vi "svx_Oct_Scale Num Plots.vi"(7 "Display State In":T1={"X Scale Width %"=50.0, "Y Scale Height %"=50.0, "X-Axis Range"={"Minimum"=0.0, "Maximum"=10.0}, "Y-Axis Range"={"Minimum"=0.0, "Maximum"=10.0}, "Z-Axis Range"={"Minimum"=0.0, "Maximum"=10.0}, "Plot Color"=0, "Frame Color"=61212, "Background Color"=16252785, "Initial AutoScale Y"=TRUE, "AutoScale X"=2, "AutoScale Y"=2, "AutoScale Z"=2, "Plot Transparency"=FALSE, "X-Axis Name"="Frequency", "Y-Axis Name"="Amplitude", "Z-Axis Name"="", "X-Axis Scaling Factor"={"Offset"=0.0, "Multiplier"=1.0}, "Y-Axis Scaling Factor"={"Offset"=0.0, "Multiplier"=1.0}, "Z-Axis Scaling Factor"={"Offset"=0.0, "Multiplier"=1.0}, "X-Scale Visible"=TRUE, "Y-Scale Visible"=TRUE, "Z-Scale Visible"=TRUE, "X-Scale Label Visible"=TRUE, "Y-Scale Label Visible"=TRUE, "Z-Scale Label Visible"=TRUE, "X-Axis Range Scaled"={"Minimum"=0.0, "Maximum"=10.0}, "Y-Axis Range Scaled"={"Minimum"=0.0, "Maximum"=10.0}, "Z-Axis Range Scaled"={"Minimum"=0.0, "Maximum"=10.0}, "Rev Z Order"=FALSE, "X-Scale Format Str"="%#.4g", "Y-Scale Format Str"="%#.4g", "Z-Scale Format Str"="%#.4g", "Decor color"=12369084, "Scale Range Change"=refnum, "out of state queue"=refnum, "property nodes"=refnum} caption="State", 11 "Waveform Array In":T2={"z0"=0.0, "dz"=1.0, "Plots"=[]} {"Plots"."Y" format="%.2f"; "Plots"."X" format="%.2f"}) -> (1 "Z length":i32, 2 "Z Index":i32, 3 "Waveform Array Out":T2={"z0"=0.0, "dz"=1.0, "Plots"=[]} {"Plots"."Y" format="%.2f"; "Plots"."X" format="%.2f"})   [LabVIEW 2017, in "SVX Octave Waterfall Graph.xctl"]
uses:
  <vilib>/addons/_XControls/Octave Waterfall Graph/SVX Octave Waterfall Graph.xctl
  <vilib>/addons/_XControls/Octave Waterfall Graph/subVIs/svx_Oct_Waterfall Data.ctl
  <vilib>/addons/_XControls/Octave Waterfall Graph/subVIs/svx_Oct_Waterfall State.ctl
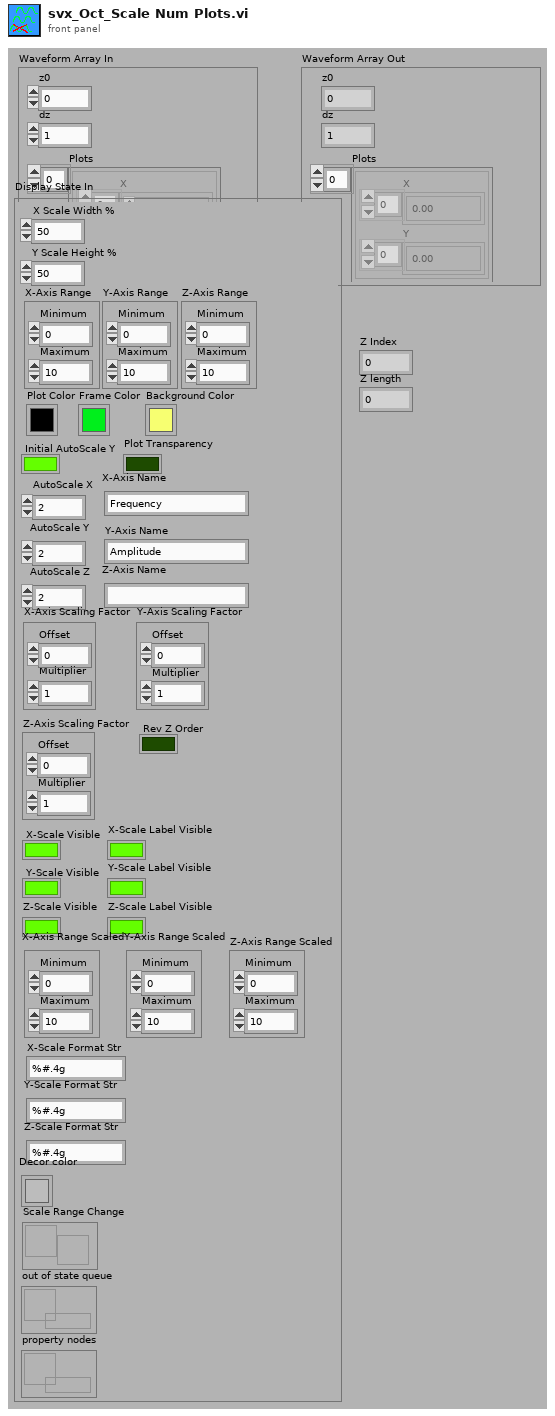
[diagram p1: front panel]
types:
  T1 = typedef "SVX Octave Waterfall Graph.xctl/svx_Oct_Waterfall State.ctl" = cluster{"X Scale Width %":dbl, "Y Scale Height %":dbl, "X-Axis Range":cluster{"Minimum":dbl, "Maximum":dbl}, "Y-Axis Range":cluster{"Minimum":dbl, "Maximum":dbl}, "Z-Axis Range":cluster{"Minimum":dbl, "Maximum":dbl}, "Plot Color":u32, "Frame Color":u32, "Background Color":u32, "Initial AutoScale Y":bool, "AutoScale X":u8, "AutoScale Y":u8, "AutoScale Z":u8, "Plot Transparency":bool, "X-Axis Name":string, "Y-Axis Name":string, "Z-Axis Name":string, "X-Axis Scaling Factor":cluster{"Offset":dbl, "Multiplier":dbl}, "Y-Axis Scaling Factor":cluster{"Offset":dbl, "Multiplier":dbl}, "Z-Axis Scaling Factor":cluster{"Offset":dbl, "Multiplier":dbl}, "X-Scale Visible":bool, "Y-Scale Visible":bool, "Z-Scale Visible":bool, "X-Scale Label Visible":bool, "Y-Scale Label Visible":bool, "Z-Scale Label Visible":bool, "X-Axis Range Scaled":cluster{"Minimum":dbl, "Maximum":dbl}, "Y-Axis Range Scaled":cluster{"Minimum":dbl, "Maximum":dbl}, "Z-Axis Range Scaled":cluster{"Minimum":dbl, "Maximum":dbl}, "Rev Z Order":bool, "X-Scale Format Str":string, "Y-Scale Format Str":string, "Z-Scale Format Str":string, "Decor color":u32, "Scale Range Change":refnum<user-event>, "out of state queue":refnum<queue>, "property nodes":refnum<queue>}
  T2 = typedef "SVX Octave Waterfall Graph.xctl/svx_Oct_Waterfall Data.ctl" = cluster{"z0":dbl, "dz":dbl, "Plots":cluster{"X":dbl[], "Y":dbl[]}[]}
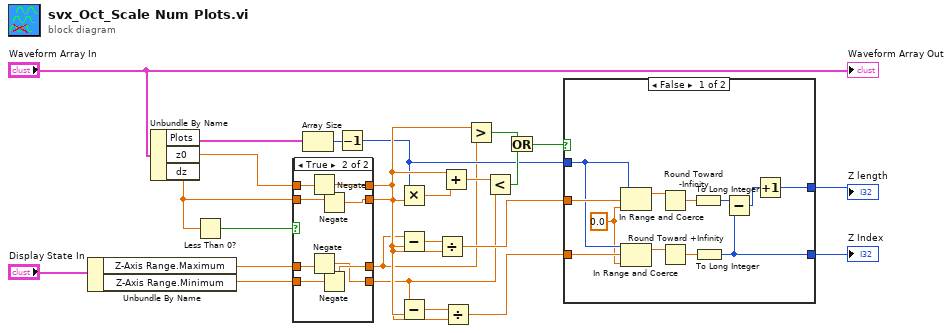
[diagram p0: block diagram]
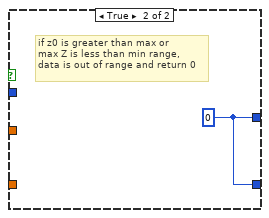
[diagram p2: hidden frame]
diagram:
  n1 = Unbundle By Name("Display State In") -> ("Z-Axis Range.Maximum"=w20:dbl, "Z-Axis Range.Minimum"=w19:dbl)
  n2 = Unbundle By Name("Waveform Array In") -> ("Plots"=w24:cluster{"X":dbl[], "Y":dbl[]}[], "z0"=w22:dbl, "dz"=w21:dbl)
  n3 = Less Than 0?(x=w21) -> (x < 0?=w23:bool)
  n4 = case shown="True" w23 {
    tunnel: w22 -> [w29 w37]
    tunnel: [w29 w36] -> w7
    tunnel: w21 -> [w28 w35]
    tunnel: [w28 w34] -> w6
    tunnel: w20 -> [w27 w33]
    tunnel: w19 -> [w26 w32]
    tunnel: [w27 w31] -> w3
    tunnel: [w26 w30] -> w2
    frame False {
    }
    frame True {
      n5 = Negate(x=w37) -> (-x=w36:dbl)
      n6 = Negate(x=w33) -> (-x=w30:dbl)
      n7 = Negate(x=w35) -> (-x=w34:dbl)
      n8 = Negate(x=w32) -> (-x=w31:dbl)
    }
  }
  n9 = Array Size(array=w24) -> (size(s)=w5:i32)
  n10 = Decrement(x=w5) -> (x-1=w4:i32)
  n11 = Multiply(x=w4, y=w6) -> (x*y=w12:dbl)
  n12 = Subtract(x=w3, y=w7) -> (x-y=w11:dbl)
  n13 = Subtract(x=w2, y=w7) -> (x-y=w10:dbl)
  n14 = Divide(x=w11, y=w6) -> (x/y=w8:dbl)
  n15 = Add(x=w7, y=w12) -> (x+y=w16:dbl)
  n16 = Divide(x=w10, y=w6) -> (x/y=w9:dbl)
  n17 = Greater?(x=w7, y=w3) -> (0:w15:bool)
  n18 = Less?(x=w16, y=w2) -> (x < y?=w14:bool)
  n19 = Or(x=w15, y=w14) -> (x .or. y?=w13:bool)
  n20 = case shown="False" w13 {
    tunnel: w8 -> [w46 _]
    tunnel: w9 -> [w45 _]
    tunnel: w4 -> [w43 _]
    tunnel: [w41 w50] -> w17
    tunnel: [w38 w50] -> w18
    frame False {
      w42 = 0.0 ("lower limit")
      n21 = In Range and Coerce(upper limit=w43, x=w46, lower limit=w42) -> (coerced(x)=w47:dbl)  [unwired: 1 out]
      n22 = In Range and Coerce(upper limit=w43, x=w45, lower limit=w42) -> (coerced(x)=w44:dbl)  [unwired: 1 out]
      n23 = Round Toward -Infinity(1:w47) -> (0:w49:dbl)
      n24 = Round Toward +Infinity(x=w44) -> (ceil(x): smallest int >= x=w40:dbl)
      n25 = To Long Integer(number=w49) -> (32bit integer=w39:i32)
      n26 = To Long Integer(number=w40) -> (32bit integer=w38:i32)
      n27 = Subtract(x=w39, y=w38) -> (x-y=w48:i32)
      n28 = Increment(x=w48) -> (x+1=w41:i32)
    }
    frame True {
      w50 = 0
      # "if z0 is greater than max or\nmax Z is less than min range,\ndata is out of range and return 0"
    }
  }
  "Z Index" <- w18
  "Z length" <- w17
  "Waveform Array Out" <- "Waveform Array In"
